vi "Connect Channels (Single).vi"(8 "error in (no error)":errorcluster, 9 "channel 2":string, 10 "channel 1":string, 11 "SLSC Switch in":refnum<class "SLSC Switch.lvclass">) -> (0 "error out":errorcluster, 3 "SLSC Switch out":refnum<class "SLSC Switch.lvclass">)   [LabVIEW 2016, in "SLSC Switch.lvlib" / "SLSC Switch.lvclass"]
doc: "Creates a path between channel 1 and channel 2. SLSC-SWITCH calculates and uses the shortest path between the two channels."
uses:
  SLSC Switch.lvclass
  SLSC Switch.lvclass/SLSC Switch.ctl
  slscsl/slscsl.lvclass
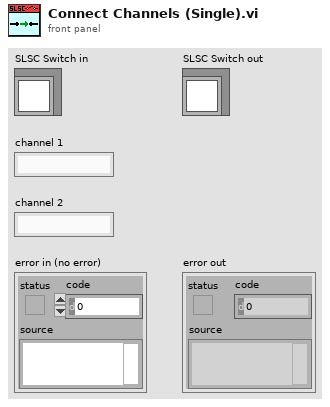
[diagram p1: front panel]
types:
  T1 = typedef "SLSC Switch.lvlib/slscsl.lvclass/SwitchActionsArray.ctl" = T2[]
  T2 = typedef "SLSC Switch.lvlib/slscsl.lvclass/SwitchAction.ctl" = cluster{"index":i32, "RelayAction":T3}
  T3 = typedef "SLSC Switch.lvlib/slscsl.lvclass/RelayAction.ctl" = u32
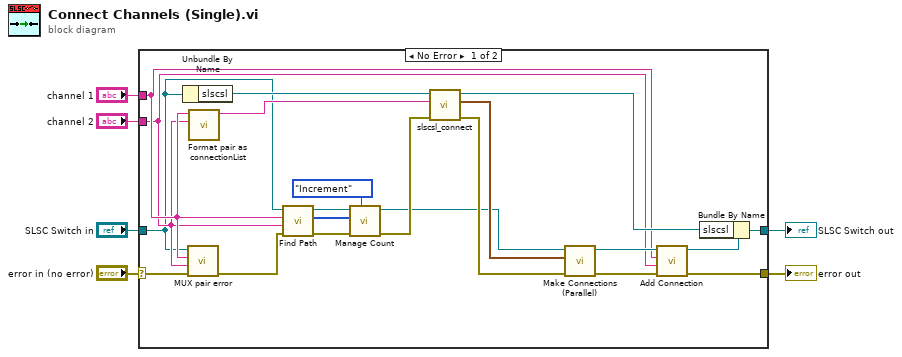
[diagram p0: block diagram]
diagram:
  n1 = case shown="No Error" "error in (no error)" {
    selector: "error in (no error)" -> [w17 w29]
    tunnel: [w22 w29] -> w5
    tunnel: "SLSC Switch in" -> [w14 w28]
    tunnel: "channel 1" -> [w16 _]
    tunnel: "channel 2" -> [w15 _]
    tunnel: [w20 w28] -> w1
    frame No Error {
      n2 = Unbundle By Name(w14) -> ("slscsl"=w26:refnum<class "slscsl.lvclass">)
      n3 = call "MUX pair error.vi"("error in (no error)"=w17, "channel 2"=w15, "channel 1"=w16, "SLSC Switch in"=w14) -> ("error out"=w10:errorcluster)  [unwired: 7 in]
      n4 = call "Format pair as connectionList.vi"("channel in"=w15, "channel 1"=w16) -> ("connectionList"=w25:string)  [unwired: 9 in]
      n5 = call "Find Path.vi"("error in (no error)"=w10, "channel 2"=w15, "channel 1"=w16, "SLSC Switch in"=w14) -> ("error out"=w11:errorcluster, "Relay Indexes"=w12:i32[], "SLSC Switch out"=w13:refnum<class "SLSC Switch.lvclass">)  [unwired: 5 in]
      n6 = call "Manage Count.vi"("Inc/Dec"=enum16{"Increment", "Decrement"}."Increment", "error in (no error)"=w11, "Relay Indexes"=w12, "SLSC Switch in"=w13) -> ("error out"=w9:errorcluster, "SLSC Switch out"=w7:refnum<class "SLSC Switch.lvclass">)  [unwired: 5 in, 1 out]
      n7 = call "slscsl_connect.vi"("error in (no error)"=w9, "connectionList"=w25, "slscsl in"=w26) -> ("error out"=w27:errorcluster, "switchActionsArray"=w18:T1, "slscsl out"=w19:refnum<class "slscsl.lvclass">)  [unwired: 6 in]
      n8 = call "Make Connections (Parallel).vi"("error in (no error)"=w27, "switchActionsArray"=w18, "SLSC Switch in"=w7) -> ("error out"=w24:errorcluster, "SLSC Switch out"=w23:refnum<class "SLSC Switch.lvclass">)  [unwired: 7 in]
      n9 = call "Add Connection.vi"("error in (no error)"=w24, "channel 2"=w15, "channel 1"=w16, "SLSC Switch in"=w23) -> ("error out"=w22:errorcluster, "SLSC Switch out"=w21:refnum<class "SLSC Switch.lvclass">)  [unwired: 6 in]
      n10 = Bundle By Name(cluster=w21, "slscsl"=w19) -> (w20:refnum<class "SLSC Switch.lvclass">)
    }
    frame Error {
    }
  }
  "error out" <- w5
  "SLSC Switch out" <- w1
